vi "start.vi"(8 "error in (no error)":errorcluster, 11 "ProEM_WinX32 in":refnum<class "ProEM_WinX32.lvclass">) -> (0 "error out":errorcluster, 3 "ProEM_WinX32 out":refnum<class "ProEM_WinX32.lvclass">)   [LabVIEW 2011, in "Hardware.lvlib" / "Channels.lvlib" / "ProEM_WinX32.lvclass"]
uses:
  ProEM_WinX32.lvclass
  ProEM_WinX32.lvclass/ProEM_WinX32.ctl
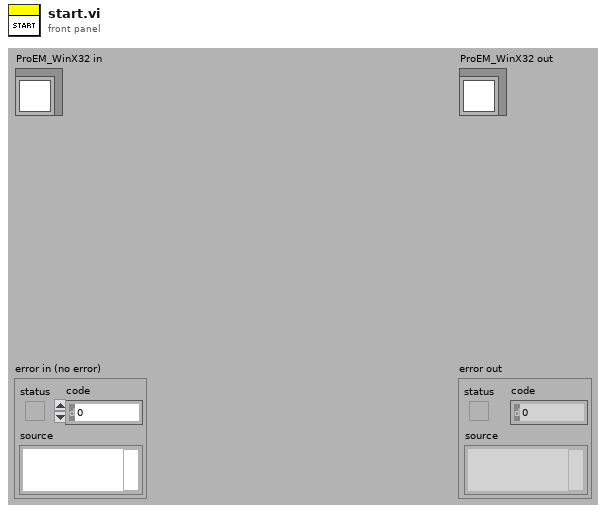
[diagram p1: front panel]
types:
  T1 = typedef "WINX32 Object Reference.ctl" = refnum<k1>
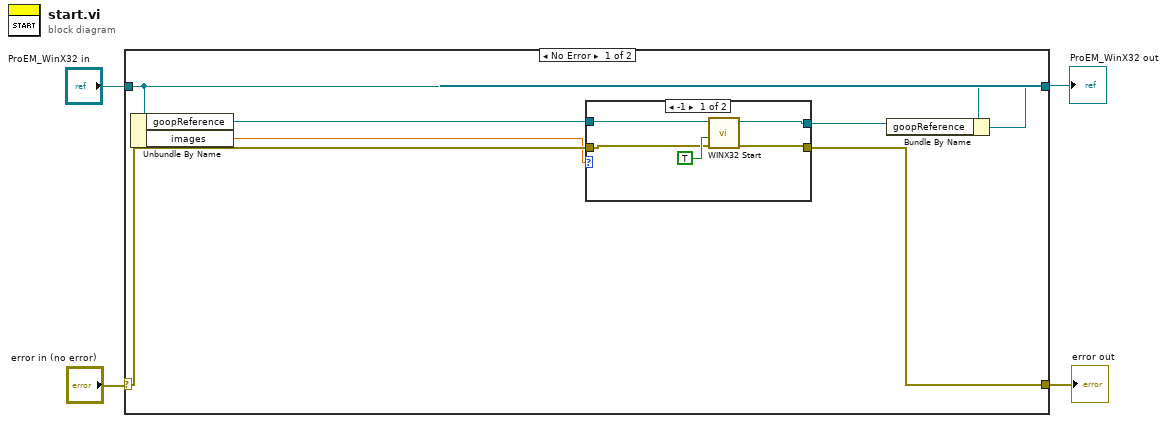
[diagram p0: block diagram]
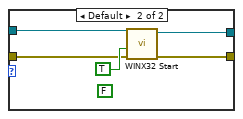
[diagram p2: hidden frame]
diagram:
  n1 = case shown="No Error" "error in (no error)" {
    selector: "error in (no error)" -> [w6 w22]
    tunnel: [w10 w23] -> w4
    tunnel: "ProEM_WinX32 in" -> [w11 w23]
    tunnel: [w8 w22] -> w1
    frame No Error {
      n2 = Unbundle By Name(w11) -> ("goopReference"=w7:T1, "images"=w5:dbl)
      n3 = case shown="-1" w5 {
        tunnel: [w14 w21] -> w9
        tunnel: [w13 w20] -> w8
        tunnel: w7 -> [w15 w18]
        tunnel: w6 -> [w12 w17]
        frame -1 {
          n4 = call <instrlib>:"WINX32 Start.vi"("error in (no error)"=w12, "Camera Active"=TRUE, "reference"=w15) -> ("error out"=w13:errorcluster, "duplicate reference"=w14:T1)  [unwired: 7 in]
        }
        frame Default {
          (unwired) FALSE
          n5 = call <instrlib>:"WINX32 Start.vi"("error in (no error)"=w17, "Camera Active"=TRUE, "reference"=w18) -> ("error out"=w20:errorcluster, "duplicate reference"=w21:T1)  [unwired: 7 in]
        }
      }
      n6 = Bundle By Name(cluster=w11, "goopReference"=w9) -> (w10:refnum<class "ProEM_WinX32.lvclass">)
    }
    frame Error {
    }
  }
  "error out" <- w1
  "ProEM_WinX32 out" <- w4
